vi "Prototype_Aug10_2016.vi"() -> ()   [LabVIEW 2015]
uses:
  <vilib>/Analysis/Matrix/Datatypes/RealMatrix.ctl
  <vilib>/Analysis/1siggen.llb/Ramp Pattern by Samples.vi
  <vilib>/Analysis/Matrix/Numeric/Conversions/Array To Matrix - RA.vi
  <vilib>/Analysis/Matrix/Numeric/Conversions/Array To Matrix - RA2.vi
  <vilib>/Analysis/Matrix/Numeric/Multiply/Multiply - RM,RM.vi
  <vilib>/Analysis/Matrix/NI_Matrix.lvlib
  <vilib>/Analysis/NI_AALBase.lvlib
panel:
  out "element":dbl
  out "appended array":T1
  out "Ramp Pattern":dbl[](array[numeric])
  out "coerced(x)":dbl[](array[numeric])
  out "number of columns":i32
  out "number of rows":i32
  out "A * B":T1
  out "Real Matrix":T1
  out "Real Matrix (Column Vector)":T1
  out "Array":dbl[](array[numeric])
  out "x^2":dbl[](array[numeric])
  out "[2]":dbl
  out "[7]":dbl
  out "[8]":dbl
  out "[0]":dbl
  out "x-y":dbl[](array[numeric])
  out "x > y?":bool[](array[boolean])
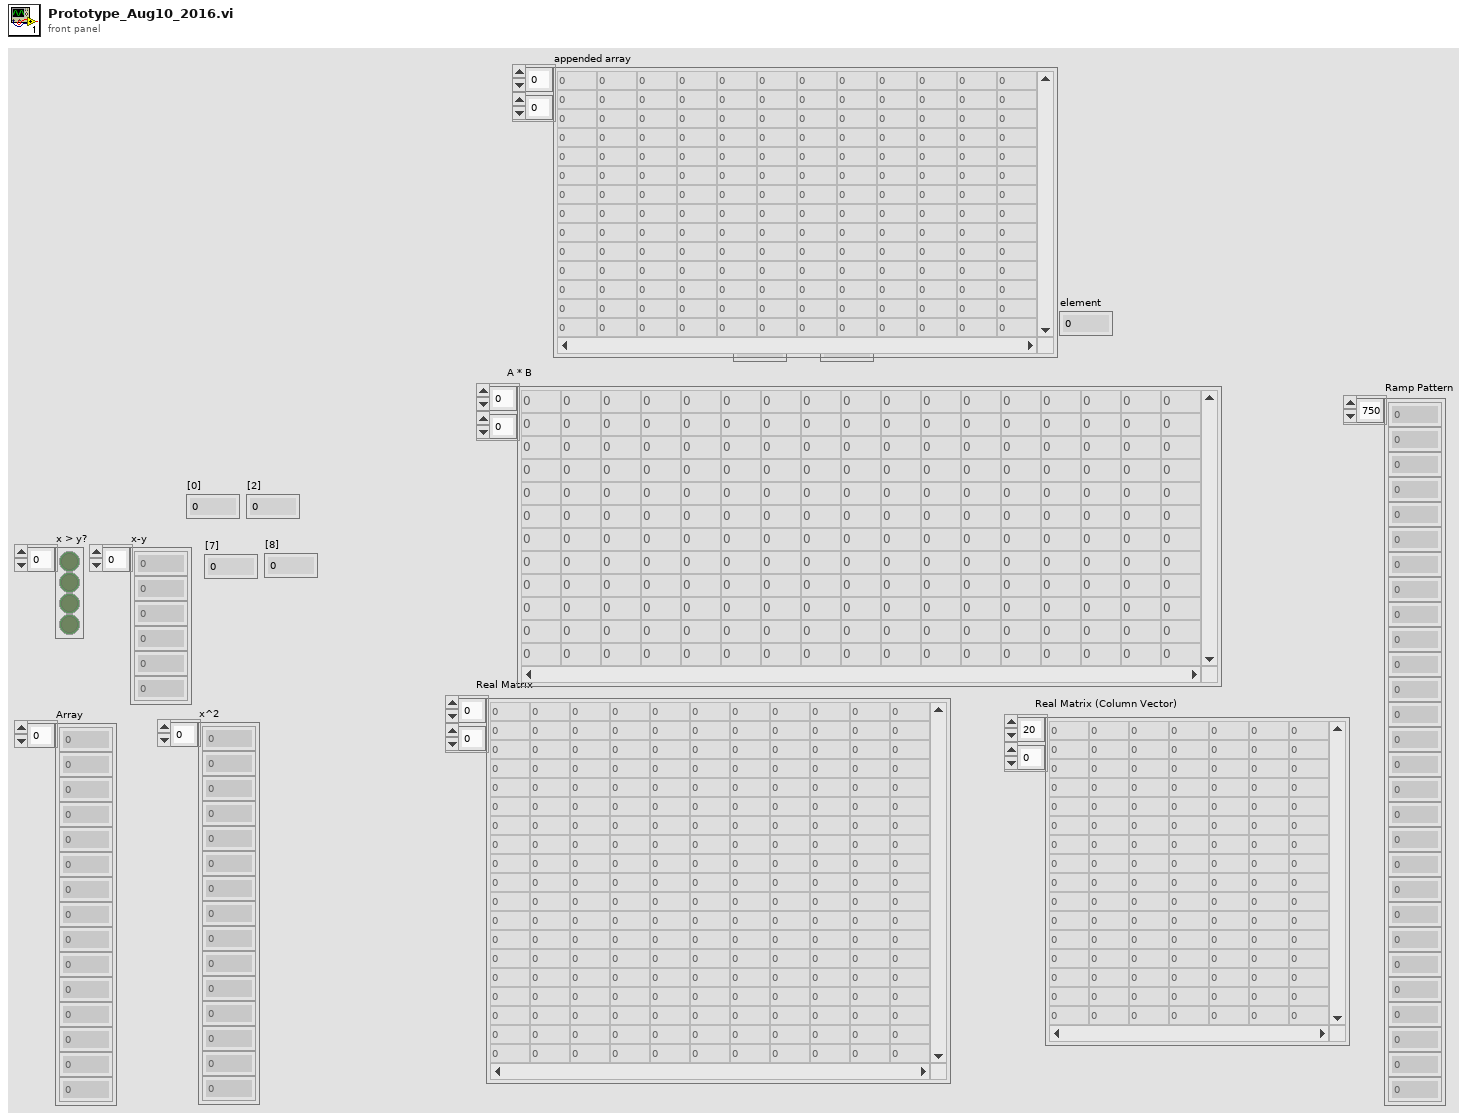
[diagram p1: front panel]
types:
  T1 = typedef "NI_Matrix.lvlib/RealMatrix.ctl" = dbl[][]
  T2 = cluster{"[0]":dbl, "[1]":dbl, "[2]":dbl, "[3]":dbl, "[4]":dbl, "[5]":dbl, "[6]":dbl, "[7]":dbl, "[8]":dbl}
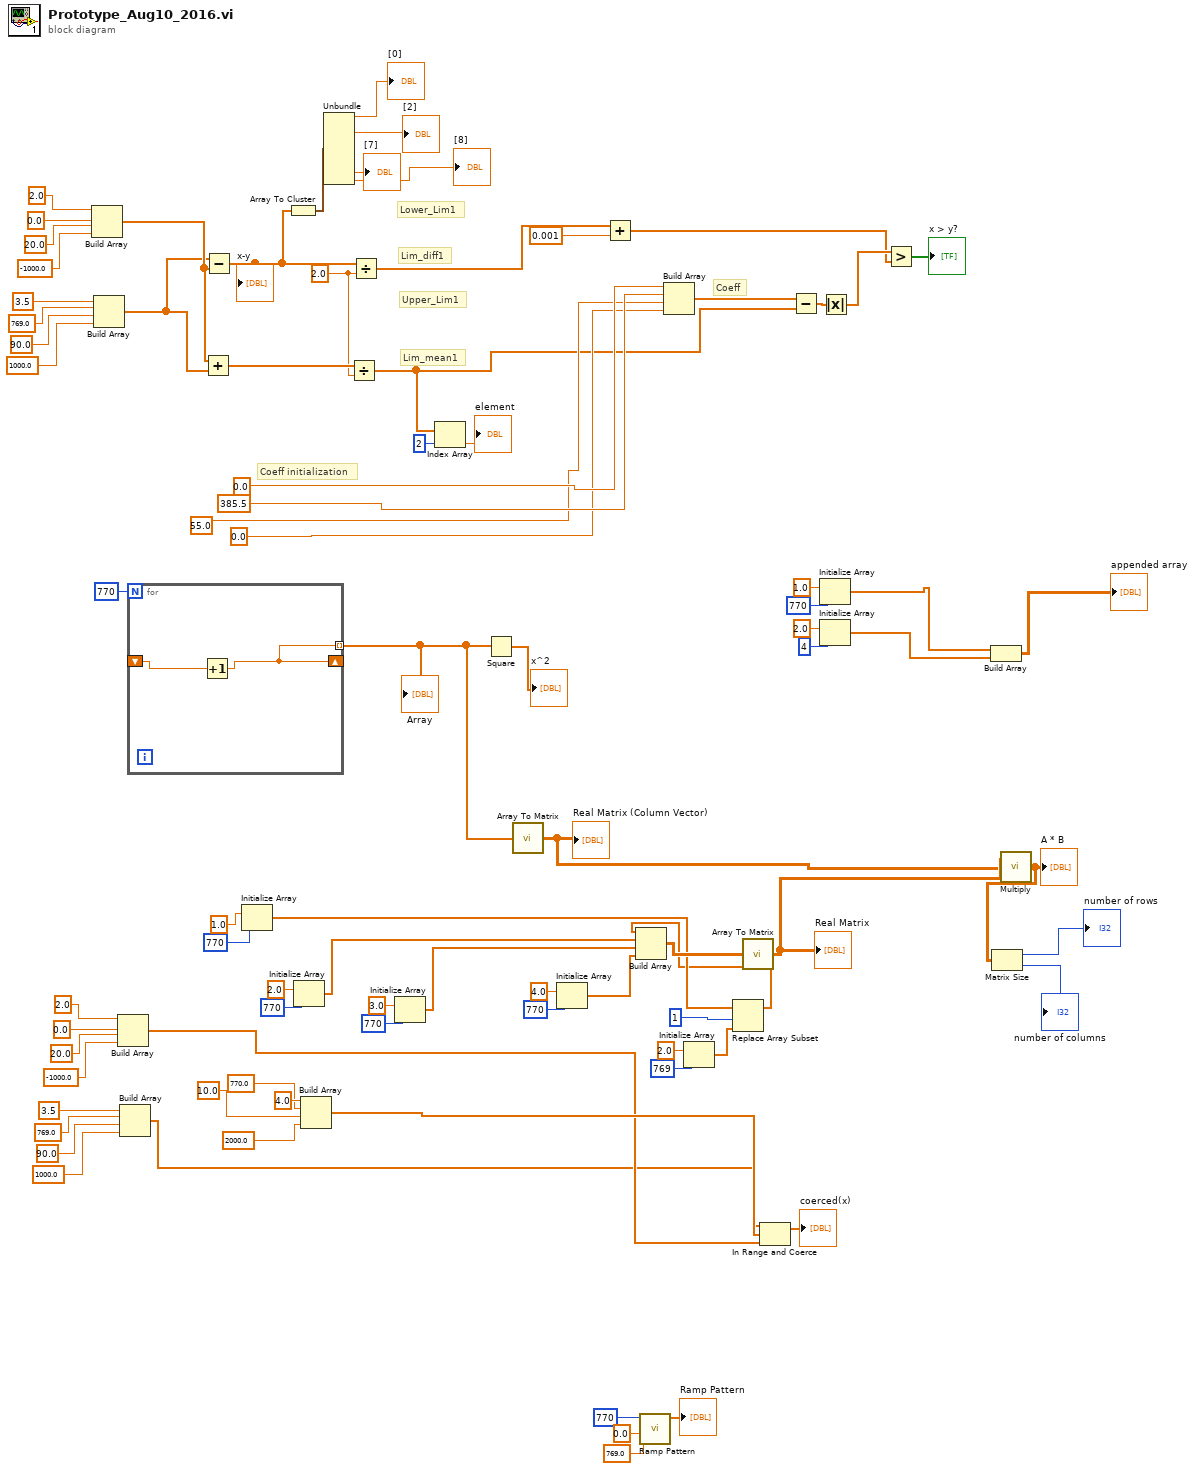
[diagram p0: block diagram]
diagram:
  w74 = 2.0 ("element")
  # "Coeff"
  # "Coeff initialization"
  # "Lim_mean1"
  # "Lim_diff1"
  # "Upper_Lim1"
  # "Lower_Lim1"
  n1 = Build Array(2.0 ("element"), 0.0 ("element"), 20.0 ("element"), -1000.0 ("element")) -> (w77:dbl[])
  n2 = Build Array(3.5 ("element"), 769.0 ("element"), 90.0 ("element"), 1000.0 ("element")) -> (w76:dbl[])
  n3 = Build Array(2.0 ("element"), 0.0 ("element"), 20.0 ("element"), -1000.0 ("element")) -> (w23:dbl[])
  n4 = Build Array(3.5 ("element"), 769.0 ("element"), 90.0 ("element"), 1000.0 ("element")) -> (w22:dbl[])
  n5 = for {
    N: 770 -> [_]
    shift-right: [w86] -> _
    shift-left: _ -> [w87]
    tunnel: [w86] -> w54 mode=indexing
    n6 = Increment(x=w87) -> (x+1=w86:dbl)
  }
  "Array" <- w54
  n7 = Add(x=w77, y=w76) -> (x+y=w75:dbl[])
  n8 = Subtract(x=w76, y=w77) -> (x-y=w62:dbl[])
  "x-y" <- w62
  n9 = Initialize Array(1.0 ("element"), 770 ("dimension size")) -> (w5:dbl[])
  n10 = Array To Cluster(array=w62) -> (cluster=w61:T2)
  n11 = Initialize Array(2.0 ("element"), 770 ("dimension size")) -> (w45:dbl[])
  n12 = Build Array(4.0 ("element"), 770.0 ("element"), 10.0 ("element"), 2000.0 ("element")) -> (w33:dbl[])
  n13 = Unbundle(w61) -> ("[0]"=→"[0]":dbl, "[2]"=→"[2]":dbl, "[7]"=→"[7]":dbl, "[8]"=→"[8]":dbl)  [unwired: 5 out]
  n14 = Divide(x=w75, y=w74) -> (x/y=w3:dbl[])
  n15 = Divide(x=w62, y=w74) -> (x/y=w68:dbl[])
  n16 = Initialize Array(3.0 ("element"), 770 ("dimension size")) -> (w44:dbl[])
  n17 = Index Array(array=w3, index=2) -> (element=→"element":dbl)
  n18 = Square(x=w54) -> (x^2=→"x^2":dbl[])
  n19 = call-poly <vilib>:"Array To Matrix.vi"("Real 1D Array"=w54) -> ("Real Matrix (Column Vector)"=w41:T1)
  "Real Matrix (Column Vector)" <- w41
  n20 = Initialize Array(4.0 ("element"), 770 ("dimension size")) -> (w43:dbl[])
  n21 = Add(x=w68, y=0.001 ("element")) -> (x+y=w69:dbl[])
  n22 = call-poly <vilib>:"Ramp Pattern.vi"("start"=0.0, "end"=769.0, "samples"=770) -> ("Ramp Pattern"=→"Ramp Pattern":dbl[])  [unwired: 7 in, 1 out]
  n23 = Build Array(0.0 ("IRQ Number(s)"), 385.5 ("IRQ Number(s)"), 55.0 ("IRQ Number(s)"), 0.0 ("IRQ Number(s)")) -> (w73:dbl[])
  n24 = Initialize Array(2.0 ("element"), 769 ("dimension size")) -> (w6:dbl[])
  n25 = Replace Array Subset(array=w5, new element=w6, index=1 ("index (row)")) -> (w4:dbl[])
  n26 = Build Array(w4, w45, w44, w43) -> (w10:dbl[][])
  n27 = call-poly <vilib>:"Array To Matrix.vi"("Real 2D Array"=w10) -> ("Real Matrix"=w42:T1)
  "Real Matrix" <- w42
  n28 = In Range and Coerce(upper limit=w22, x=w33, lower limit=w23) -> (coerced(x)=→"coerced(x)":dbl[])  [unwired: 1 out]
  n29 = Subtract(x=w73, y=w3) -> (x-y=w72:dbl[])
  n30 = Initialize Array(1.0 ("element"), 770 ("dimension size")) -> (w13:dbl[])
  n31 = Initialize Array(2.0 ("element"), 4 ("dimension size")) -> (w12:dbl[])
  n32 = Absolute Value(x=w72) -> (abs(x)=w71:dbl[])
  n33 = Greater?(x=w71, y=w69) -> (0:→"x > y?":bool[])
  n34 = Build Array(w13, w12) -> (→"appended array":dbl[][])
  n35 = call-poly <vilib>:"Multiply.vi"("Real Matrix B"=w41, "Real Matrix A"=w42) -> ("A * B"=w40:T1)
  "A * B" <- w40
  n36 = Matrix Size(0:w40) -> (1:→"number of rows":i32, 2:→"number of columns":i32)
